vi "Quizz7.vi"() -> ()   [LabVIEW 2017]
panel:
  out "Numeric 4":dbl
  out "Numeric 3":dbl
  out "Numeric 2":dbl
  out "x*y 2":i8
  out "Boolean 2":bool
  out "x+y 2":dbl
  out "Boolean":bool
  out "x*y":i8
  out "Numeric":dbl
  out "x+y":dbl
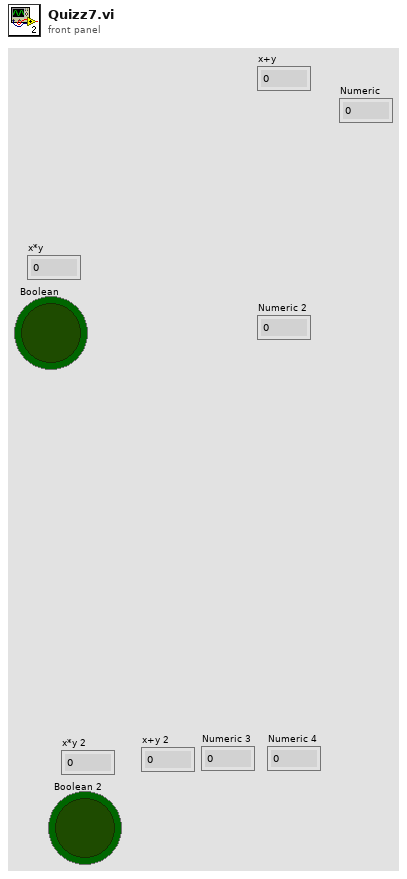
[diagram p1: front panel]
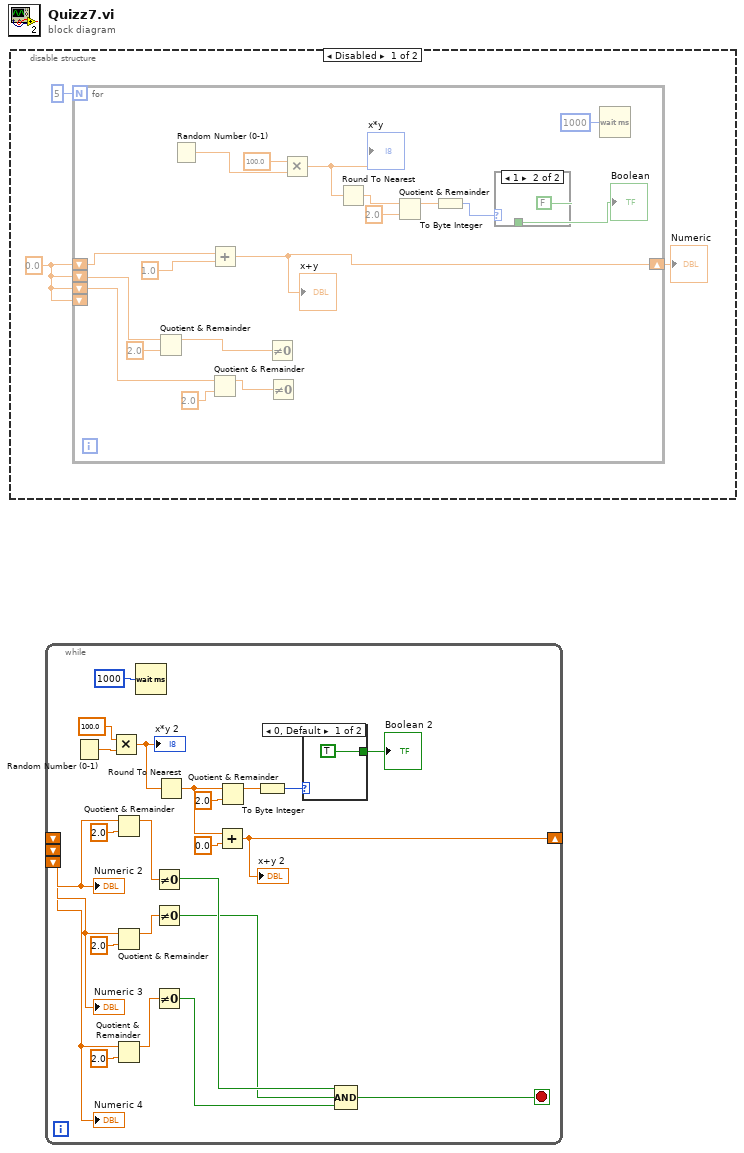
[diagram p0: block diagram]
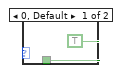
[diagram p2: hidden frame]
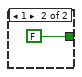
[diagram p4: hidden frame]
diagram:
  n1 = disable-structure shown="Disabled" {
    frame Disabled {
      w2 = 0.0
      n2 = for {
        N: 5 -> [_]
        shift-right: [w16] -> w1
        shift-left: w2 -> [w19]
        shift-left: w2 -> [w18]
        shift-left: w2 -> [w17]
        shift-left: w2 -> [_]
        n3 = Quotient & Remainder(x=w18, y=2.0) -> (x-y*floor(x/y)=w7:dbl)  [unwired: 1 out]
        n4 = Random Number (0-1)() -> (number: 0 to 1=w15:dbl)
        n5 = Add(x=w19, y=1.0) -> (x+y=w16:dbl)
        "x+y" <- w16
        n6 = Quotient & Remainder(x=w17, y=2.0) -> (x-y*floor(x/y)=w4:dbl)  [unwired: 1 out]
        n7 = Not Equal To 0?(x=w7) -> ()  [unwired: 1 out]
        n8 = Not Equal To 0?(x=w4) -> ()  [unwired: 1 out]
        n9 = Multiply(x=100.0, y=w15) -> (x*y=w11:dbl)
        "x*y" <- w11
        n10 = Round To Nearest(number=w11) -> (nearest integer value=w10:dbl)
        n11 = Quotient & Remainder(x=w10, y=2.0) -> (x-y*floor(x/y)=w8:dbl)  [unwired: 1 out]
        n12 = To Byte Integer(number=w8) -> (8bit integer=w13:i8)
        n13 = case shown="1" w13 {
          tunnel: [TRUE FALSE] -> w12
          frame 0, Default {
          }
          frame 1 {
          }
        }
        "Boolean" <- w12
        n14 = Wait (ms)(milliseconds to wait=u32 1000) -> ()  [unwired: 1 out]
      }
      "Numeric" <- w1
    }
    frame Enabled {
    }
  }
  n15 = while {
    shift-right: [w42] -> _
    shift-left: _ -> [w26]
    shift-left: _ -> [w25]
    shift-left: _ -> [w24]
    stop <- w28 stop-if-true
    n16 = Random Number (0-1)() -> (number: 0 to 1=w32:dbl)
    n17 = Multiply(x=100.0, y=w32) -> (x*y=w34:dbl)
    "x*y 2" <- w34
    n18 = Quotient & Remainder(x=w26, y=2.0) -> (x-y*floor(x/y)=w44:dbl)  [unwired: 1 out]
    n19 = Quotient & Remainder(x=w25, y=2.0) -> (x-y*floor(x/y)=w47:dbl)  [unwired: 1 out]
    n20 = Quotient & Remainder(x=w24, y=2.0) -> (x-y*floor(x/y)=w38:dbl)  [unwired: 1 out]
    n21 = Wait (ms)(milliseconds to wait=u32 1000) -> ()  [unwired: 1 out]
    n22 = Not Equal To 0?(x=w44) -> (x != 0?=w41:bool)
    n23 = Not Equal To 0?(x=w47) -> (x != 0?=w40:bool)
    n24 = Not Equal To 0?(x=w38) -> (x != 0?=w37:bool)
    n25 = Round To Nearest(number=w34) -> (nearest integer value=w27:dbl)
    n26 = Add(x=w27, y=0.0) -> (x+y=w42:dbl)
    "x+y 2" <- w42
    n27 = Quotient & Remainder(x=w27, y=2.0) -> (x-y*floor(x/y)=w36:dbl)  [unwired: 1 out]
    n28 = To Byte Integer(number=w36) -> (8bit integer=w30:i8)
    n29 = case shown="0, Default" w30 {
      tunnel: [TRUE FALSE] -> w29
      frame 0, Default {
      }
      frame 1 {
      }
    }
    "Boolean 2" <- w29
    n30 = Compound Arithmetic op=AND(w41, w40, w37) -> (w28:bool)
    "Numeric 2" <- w26
    "Numeric 3" <- w25
    "Numeric 4" <- w24
  }
